vi "Tosca-Create Raw Data File.vi"(0 "refnum in":refnum<file>, 1 "Length":i32, 2 "Remainder":dbl[][](array[numeric]), 5 "Filestem":string, 7 "Header":string, 9 "Trial Number":i32, 11 "error in":errorcluster) -> (4 "refnum out":refnum<file>, 15 "error out":errorcluster)   [LabVIEW 2020]
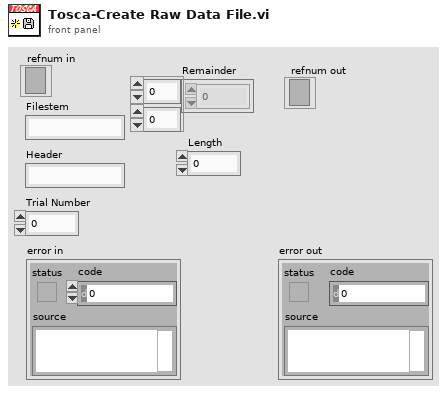
[diagram p1: front panel]
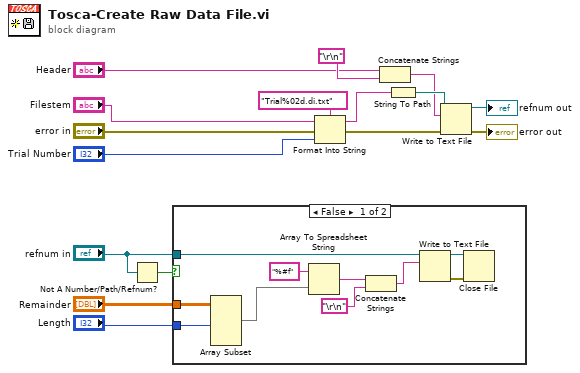
[diagram p0: block diagram]
diagram:
  n1 = Not A Number/Path/Refnum?(number/path/refnum="refnum in") -> (NaN/Path/Refnum?=w7:bool)
  n2 = case shown="False" w7 {
    tunnel: "refnum in" -> [w24 _]
    tunnel: "Remainder" -> [w22 _]
    tunnel: "Length" -> [w21 _]
    frame False {
      n3 = Array Subset(array=w22, length (row)=w21) -> (w20:dbl[][])  [unwired: 3 in]
      n4 = Array To Spreadsheet String(array=w20, 3:"%#f" ("format string")) -> (spreadsheet string=w19:string)  [unwired: 1 in]
      n5 = Concatenate Strings(w19, "\r\n") -> (w17:string)
      n6 = Write to Text File(file (use dialog)=w24, text=w17) -> (refnum out=w25:refnum<file>, error out=w26:errorcluster)  [unwired: 2 in, 1 out]
      n7 = Close File(refnum=w25, error in=w26) -> ()  [unwired: 2 out]
    }
    frame True {
    }
  }
  n8 = Format Into String(format string="Trial%02d.di.txt", initial string="Filestem", error in="error in", "Trial Number") -> (resulting string=w15:string, error out=w13:errorcluster)
  n9 = Concatenate Strings("Header", "\r\n") -> (w10:string)
  n10 = String To Path(string=w15) -> (path=w14:path)
  n11 = Write to Text File(file (use dialog)=w14, text=w10, error in=w13) -> (refnum out=→"refnum out":refnum<file>, error out=→"error out":errorcluster)  [unwired: 1 in, 1 out]
